vi "Write.vi"(6 "Append Index":i32, 8 "error in (no error)":errorcluster, 9 "Notes":string, 10 "Data (Dictionary)":T1[](array[typedef]), 11 "Data.ITX in":refnum<class "Data.ITX.lvclass">) -> (0 "error out":errorcluster, 3 "Data.ITX out":refnum<class "Data.ITX.lvclass">, 5 "Path out":path)   [LabVIEW 2019, in "Data.ITX.lvclass"]
uses:
  Data.ITX.lvclass
  Data/Data.lvclass
  ITX Commands/ITX Commands.lvclass
  Data/Typedefs/Dictionary--cluster.ctl
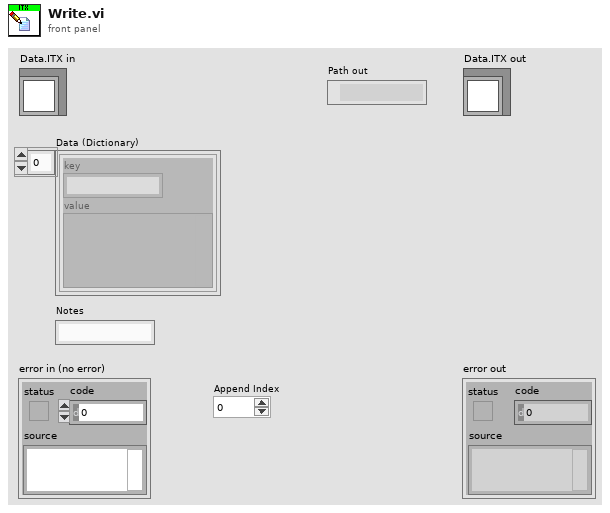
[diagram p1: front panel]
types:
  T1 = typedef "Data.lvclass/Dictionary--cluster.ctl" = cluster{"key":string, "value":variant}
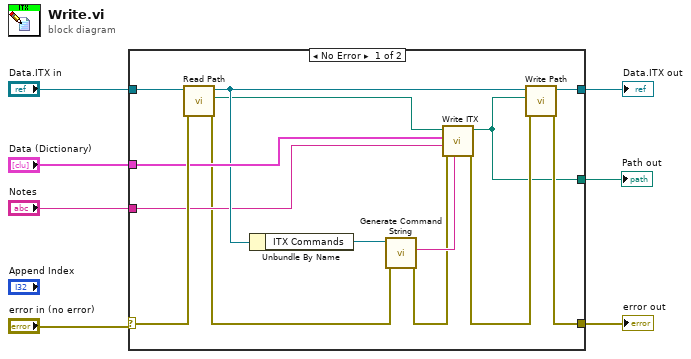
[diagram p0: block diagram]
diagram:
  n1 = case shown="No Error" "error in (no error)" {
    selector: "error in (no error)" -> [w20 w23]
    tunnel: [w18 w23] -> w4
    tunnel: "Data.ITX in" -> [w21 w22]
    tunnel: [w19 w22] -> w5
    tunnel: "Data (Dictionary)" -> [w16 _]
    tunnel: "Notes" -> [w12 _]
    tunnel: [w8 _] -> w1
    frame No Error {
      n2 = call "Read Path.vi"("error in (no error)"=w20, "Data Save"=w21) -> ("error out"=w11:errorcluster, "Path"=w9:path, "Data Save out"=w15:refnum<class "Data.ITX.lvclass">)  [unwired: 7 in]
      n3 = Unbundle By Name(w15) -> ("ITX Commands"=w14:refnum<class "ITX Commands.lvclass">)
      n4 = call "Generate Command String.vi"("ITX Commands in"=w14, "error in (no error)"=w11) -> ("ITX Commands"=w13:string, "error out"=w10:errorcluster)  [unwired: 6 in, 1 out]
      n5 = call "Write ITX.vi"("Commands"=w13, "error in"=w10, "Notes"=w12, "Data (Dictionary)"=w16, "filename"=w9) -> ("error out"=w17:errorcluster, "file"=w8:path)  [unwired: 5 in]
      n6 = call "Write Path.vi"("error in (no error)"=w17, "Path"=w8, "Data Save"=w15) -> ("error out"=w18:errorcluster, "Data Save out"=w19:refnum<class "Data.ITX.lvclass">)  [unwired: 7 in]
    }
    frame Error {
    }
  }
  "error out" <- w4
  "Data.ITX out" <- w5
  "Path out" <- w1
